vi "gxml_DuplicateTagChk.vi"(7 "error in":errorcluster, 10 "Cluster Elements":variant[](array[variant])) -> (0 "error out":errorcluster, 3 "Cluster Elements Out":variant[](array[variant]))   [LabVIEW 2011, in "Third Party VIs.lvlib" / "GXML.lvlib"]
doc: "Ensures no two elements of the same hierarchy have the same name."
uses:
  GXML.lvlib
  <vilib>/Utility/VariantDataType/VariantType.lvlib
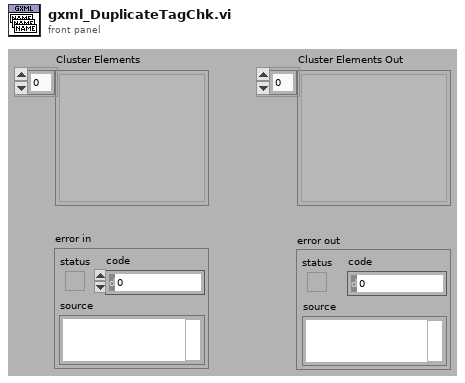
[diagram p1: front panel]
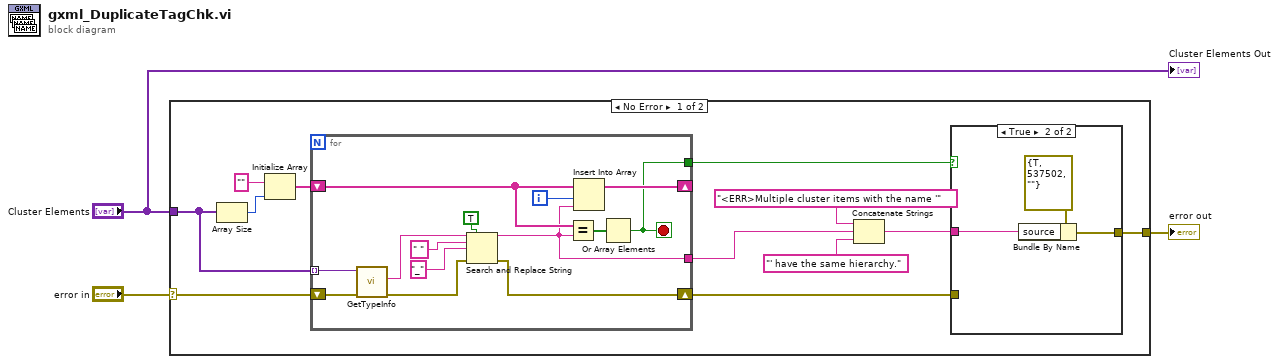
[diagram p0: block diagram]
diagram:
  n1 = case shown="No Error" "error in" {
    selector: "error in" -> [w4 w34]
    tunnel: "Cluster Elements" -> [w14 _]
    tunnel: [w5 w34] -> w2
    frame No Error {
      n2 = Array Size(array=w14) -> (size(s)=w13:i32)
      n3 = Initialize Array("", w13) -> (w12:string[])
      n4 = for {
        tunnel: w14 -> [w33] mode=indexing
        shift-right: [w26] -> w6
        shift-left: w4 -> [w32]
        shift-right: [w25] -> _
        shift-left: w12 -> [w23]
        tunnel: [w21] -> w9
        tunnel: [w20] -> w7
        i -> [w24]
        stop <- w20 stop-if-true
        n5 = call <vilib>:"GetTypeInfo.vi"("error in (no error)"=w32, "Variant"=w33) -> ("error out"=w27:errorcluster, "Name"=w28:string)  [unwired: 5 in, 3 out]
        n6 = Search and Replace String(replace all?=TRUE ("replace all? (F)"), input string=w28, search string=" " ("regular expression (\"\")"), replace string="_" ("replace string (\"\")"), error in=w27) -> (result string=w21:string, error out=w26:errorcluster)  [unwired: 3 in, 2 out]
        n7 = Equal?(x=w23, y=w21) -> (x = y?=w22:bool[])
        n8 = Insert Into Array(array=w23, index=w24, new element=w21) -> (w25:string[])
        n9 = Or Array Elements(Boolean array=w22) -> (logical OR=w20:bool)
      }
      n10 = Concatenate Strings("<ERR>Multiple cluster items with the name '", w9, "' have the same hierarchy.") -> (w11:string)
      n11 = case shown="True" w7 {
        tunnel: w6 -> [w16 _]
        tunnel: [w16 w18] -> w5
        tunnel: w11 -> [_ w17]
        frame False {
        }
        frame True {
          n12 = Bundle By Name(cluster=errorcluster {"status"=TRUE, "code"=537502, "source"=""} ("error in"), "source"=w17) -> (w18:errorcluster)
        }
      }
    }
    frame Error {
    }
  }
  "error out" <- w2
  "Cluster Elements Out" <- "Cluster Elements"
